vi "Angle Processing Unit - Multi FPGA.vi"(6 "trigger line.<user name>":refnum<k21>="PXI_Trig0", 7 "settings.<user name>":T4, 8 "register bus":T2={"Speed"="Speed", "Crank Angle"="Crank Angle", "Cycle Angle"="Cycle Angle", "Crank Count"="Crank Count", "Cycle Count"="Cycle Count", "1.25 MHz Counter"="1.25 MHz Counter", "Crank Rollover"="Crank Rollover", "Cycle Rollover"="Cycle Rollover", "shared settings"={"start"=0.0, "stuck limit"=0.0}} {"shared settings"."start" format="%#.15g"}, 9 "master":bool, 11 "input.<user name>":T1={"desired speed"=0.0, "reset"=TRUE}) -> (3 "output.<user name>":T5)   [LabVIEW 2015, in "Engine Simulation Toolkit.lvlib" / "APU.lvlib"]
doc: "Simulates a rotating engine with speed and (optionally) acceleration and publishes crank and cycle positions to the register bus. <b> This VI should be in an SCTL</b>. Use this VI when synchronizing a single APU across multiple FPGAs. It will keep all inputs and output synchronized.\n\n<b>settings.<user name></b> - settings for the component. NI VeriStand will set these values. Create a control for this input. Replace <user name> with the name you wish this component to display as inside NI VeriStand. Make this name consistent for all controls, indicators, for all VIs of this component.\n<b>input.<user name></b> - input for the component. NI VeriStand will set these values. Create a control for this input. Replace <user name> with the name you wish this component to display as inside NI VeriStand. Make this name consistent for all controls, indicators, for all VIs of this component.\n<b>sync.<user name></b> - starts a synchronization pulse. NI VeriStand will set this value. Create a control for this input and make sure the mechanical action is Latch When Released. Replace <user name> with the name you wish this component to display as inside NI VeriStand. Make this name consistent for all controls, indicators, for all VIs of this component.\n<b>trigger line.<user name></b> - connect this input to the output of the initialize APU VI. This contains a reference to the synchronization trigger line.\n<b>register bus</b> - connect this input to the output of the initialize APU VI. This contains references to APU state variables like position and speed.\n\n<b>output.<user name></b> - output for the component. NI VeriStand will read these values. Create an indicator for this output. Replace <user name> with the name you wish this component to display as inside NI VeriStand. Make this name consistent for all controls, indicators, for all VIs of this component."
uses:
  APU.lvlib
  Output.ctl
  Settings.ctl
  Register Bus.ctl
  Shared Settings.ctl
  Input.ctl
  <vilib>/rvi/eio/common/nirviEmuTemplateMethod_errors.vi
  <vilib>/eio/EIONode/EIONode.xnode
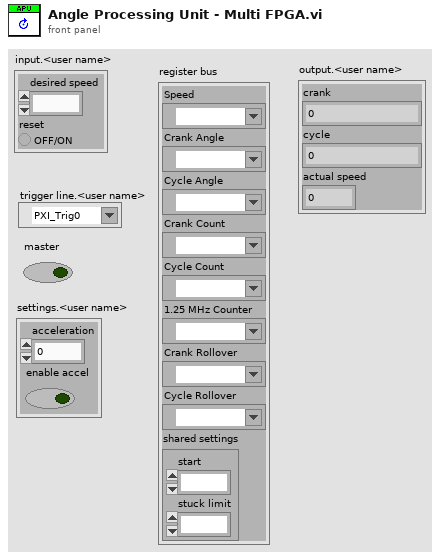
[diagram p1: front panel]
types:
  T1 = typedef "Engine Simulation Toolkit.lvlib/APU.lvlib/Input.ctl" = cluster{"desired speed":fxp<+/-,23,2>, "reset":bool}
  T2 = typedef "Engine Simulation Toolkit.lvlib/APU.lvlib/Register Bus.ctl" = cluster{"Speed":refnum<k21>, "Crank Angle":refnum<k21>, "Cycle Angle":refnum<k21>, "Crank Count":refnum<k21>, "Cycle Count":refnum<k21>, "1.25 MHz Counter":refnum<k21>, "Crank Rollover":refnum<k21>, "Cycle Rollover":refnum<k21>, "shared settings":T3}
  T3 = typedef "Engine Simulation Toolkit.lvlib/APU.lvlib/Shared Settings.ctl" = cluster{"start":fxp<+,17,17>, "stuck limit":fxp<+,18,18>}
  T4 = typedef "Engine Simulation Toolkit.lvlib/APU.lvlib/Settings.ctl" = cluster{"acceleration":fxp<+,18,-20>, "enable accel":bool}
  T5 = typedef "Engine Simulation Toolkit.lvlib/APU.lvlib/Output.ctl" = cluster{"crank":u16, "cycle":u16, "actual speed":fxp<+/-,23,2>}
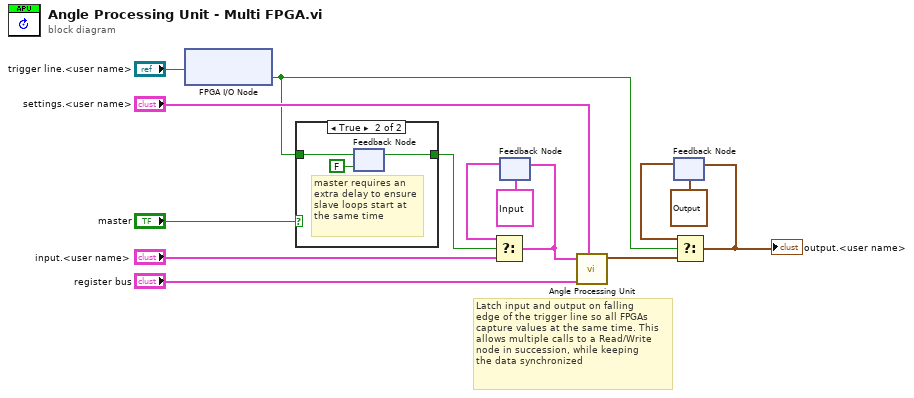
[diagram p0: block diagram]
diagram:
  # "Latch input and output on falling\nedge of the trigger line so all FPGAs\ncapture values at the same time. This\nallows multiple calls to a Read/Write\nnode in succession, while keeping\nthe data synchronized"
  n1 = xnode "FPGA I/O Node"("FPGA I/O In"="trigger line.<user name>") -> ("I/O Item"=w2:bool)  [unwired: 1 out]
  n2 = case shown="True" "master" {
    tunnel: w2 -> [w15 w18]
    tunnel: [w15 w16] -> w1
    frame False {
    }
    frame True {
      # "master requires an\nextra delay to ensure\nslave loops start at\nthe same time"
      n3 = feedback-in #1(w18) -> ()
      n4 = feedback #1(FALSE ("I/O Item")) -> (w16:bool)
    }
  }
  n5 = feedback #2(T1 {"desired speed"=0.0, "reset"=TRUE} ("input.<user name>")) -> (w10:T1)
  n6 = Select(t=w10, s=w1, f="input.<user name>") -> (s? t:f=w9:T1)
  n7 = feedback-in #2(w9) -> ()
  n8 = call "Angle Processing Unit.vi"("settings.<user name>"="settings.<user name>", "register bus"="register bus", "input.<user name>"=w9) -> ("output.<user name>"=w7:T5)  [unwired: 8 in]
  n9 = feedback #3(T5 {"crank"=0, "cycle"=0, "actual speed"=0.0} ("output.<user name>")) -> (w6:T5)
  n10 = Select(t=w6, s=w2, f=w7) -> (s? t:f=w5:T5)
  "output.<user name>" <- w5
  n11 = feedback-in #3(w5) -> ()
